vi "SaveTestTreeAs.vi"(7 "Action":T2, 8 "error in (no error)":errorcluster, 10 ".tst File Path":path, 11 "ListboxRef":refnum<vi>) -> (0 "error out":errorcluster, 1 "Cancelled?":bool, 2 "path.tstFile":path, 3 "All Test Tree Tags":string[](array[string]), 4 "Test Configuration":T1)   [LabVIEW 2018]
uses:
  TestConfigurationActions.ctl
  TestConfiguration.ctl
  <vilib>/Utility/config.llb/NI_LVConfig.lvlib
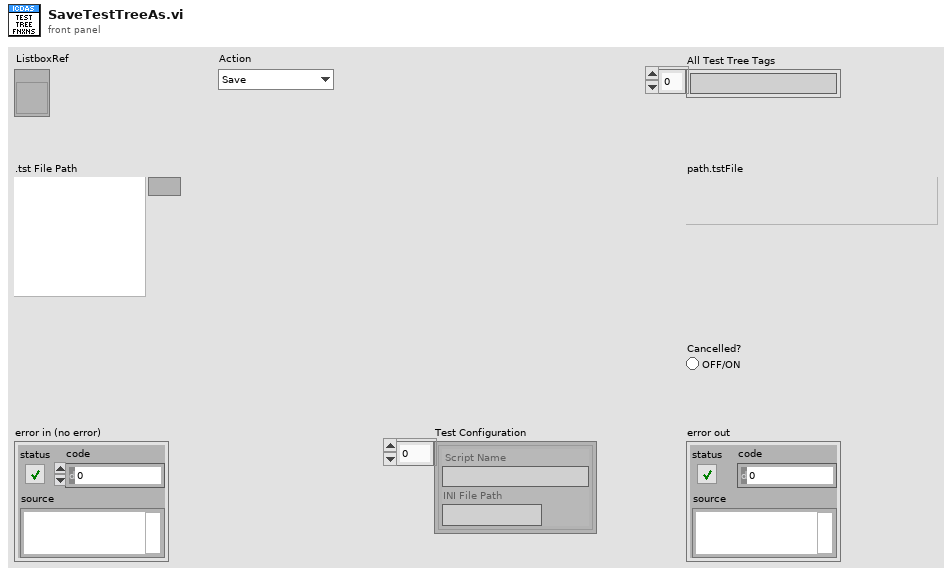
[diagram p1: front panel]
types:
  T1 = typedef "TestConfiguration.ctl" = cluster{"Script Name":string, "INI File Path":string}[]
  T2 = typedef "TestConfigurationActions.ctl" = enum16{"Save", "Save As", "Read", "Read&Load"}
  T3 = typedef "NI_LVConfig.lvlib/Config Data RefNum.ctl" = refnum<k1>
  T4 = typedef "cntlRefs.ctl" = cluster{"rngFGen":refnum<vi>, "rngDigitizer":refnum<vi>, "btnHide":refnum<vi>, "rngInst":refnum<vi>, "Instrument Modules":refnum<vi>, "RelativePathToINIFiles ":refnum<vi>, "PluginTree":refnum<vi>, "TestListboxRef":refnum<vi>, "path.tstFile":refnum<vi>, "cmbxRunningModules":refnum<vi>, "TestDataSubPanel":refnum<vi>, "TestDataCaption":refnum<vi>, "btnPopInOut":refnum<vi>, "PluginMgrQ":refnum<queue>, "TestMgrQ":refnum<queue>, "TestMgrSubPanel":refnum<vi>, "PluginMgrSubPanel":refnum<vi>, "PwrReqHandle":u32, "btnStopOneTest":refnum<vi>, "pathUserfiles":refnum<vi>}
  T5 = cluster{"Script Name":string, "INI File Path":string}
  T6 = typedef "Plugin Tree Tag.ctl" = cluster{"ItemType":T7, "Name":string, "Path":path, "Script":string[]}
  T7 = typedef "Plugins Tree Item Type.ctl" = enum16{"Plugin", "Instrument", "INI File", "INI Script"}
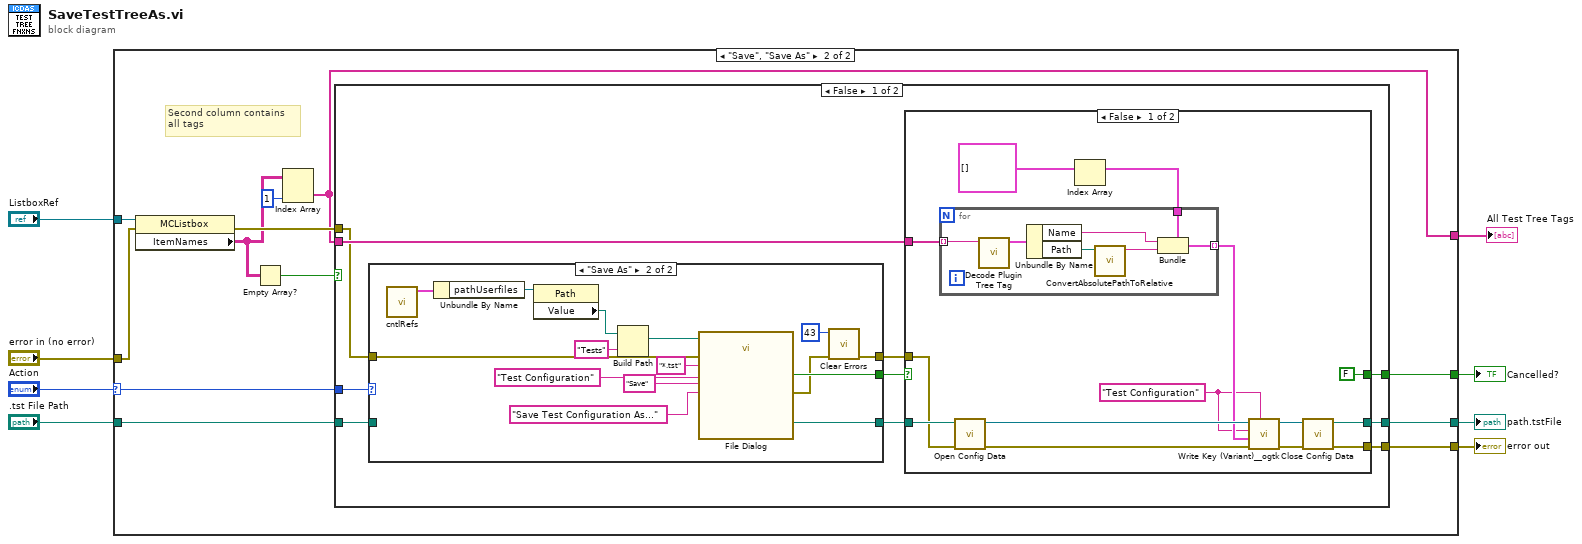
[diagram p0: block diagram]
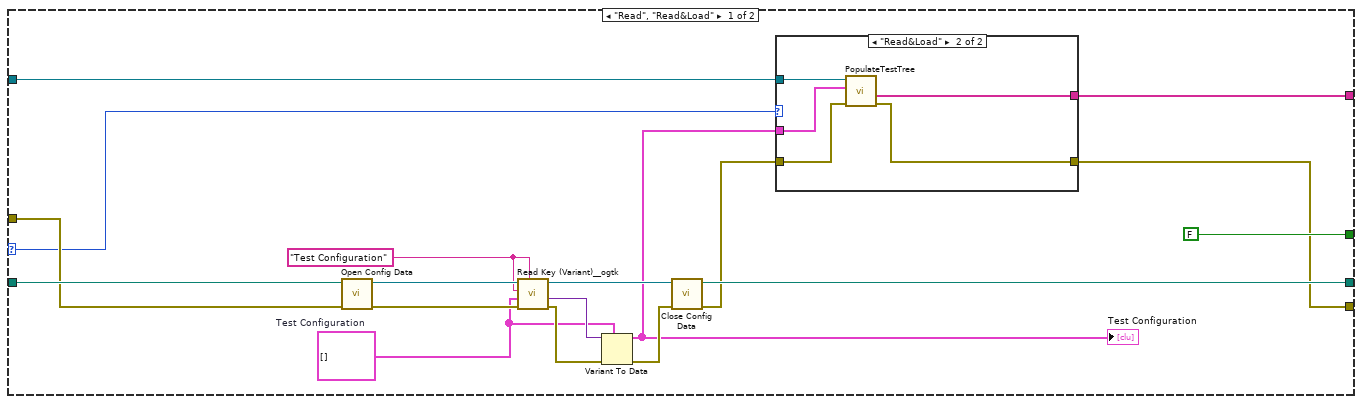
[diagram p2: hidden frame]
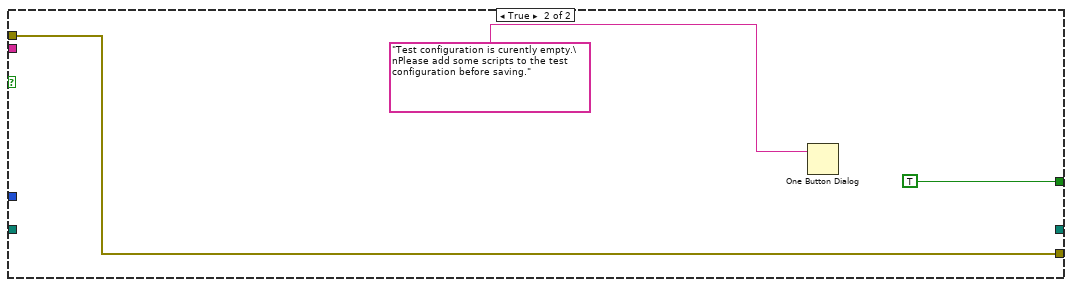
[diagram p6: hidden frame]
diagram:
  n1 = case shown="\"Save\", \"Save As\"" "Action" {
    selector: "Action" -> [w14 w40]
    tunnel: "ListboxRef" -> [w13 w43]
    tunnel: "error in (no error)" -> [w25 w42]
    tunnel: [w11 w39] -> w2
    tunnel: [FALSE w38] -> w5
    tunnel: [w18 w37] -> w4
    tunnel: ".tst File Path" -> [w26 w36]
    tunnel: [w9 w33] -> w1
    frame "Read", "Read&Load" {
      w15 = "Test Configuration" ("section")
      w21 = T1 []  # Test Configuration
      n2 = call <vilib>:"Open Config Data.vi"("error in (no error)"=w25, "configuration file path"=w26) -> ("error out"=w24:errorcluster, "refnum"=w16:T3)  [unwired: 7 in, 1 out]
      n3 = call <userlib>:"Read Key (Variant)__ogtk.vi"("section"=w15, "error in (no error)"=w24, "type"=w21, "key (optional)"=w15, "refnum"=w16) -> ("error out"=w22:errorcluster, "key-value"=w23:variant, "refnum out"=w19:T3)  [unwired: 3 in, 1 out]
      n4 = Variant To Data(error in=w22, type=w21, Variant=w23) -> (data=w10:T1, error out=w20:errorcluster)
      "Test Configuration" <- w10
      n5 = call <vilib>:"Close Config Data.vi"("error in (no error)"=w20, "refnum"=w19) -> ("error out"=w12:errorcluster, "file path"=w18:path)  [unwired: 8 in]
      n6 = case shown="\"Read&Load\"" w14 {
        tunnel: w13 -> [_ w32]
        tunnel: w10 -> [_ w31]
        tunnel: w12 -> [w27 w29]
        tunnel: [w27 w30] -> w11
        tunnel: [_ w28] -> w9
        frame Default {
        }
        frame "Read&Load" {
          n7 = call "PopulateTestTree.vi"("error in (no error)"=w29, "Test Configuration"=w31, "ListboxRef"=w32) -> ("error out"=w30:errorcluster, "All Test Tree Tags"=w28:string[])  [unwired: 7 in]
        }
      }
    }
    frame "Save", "Save As" {
      # "Second column contains\nall tags"
      n8 = property class="MCListbox"(reference=w43, error in=w42) -> (error out=w41:errorcluster, "ItemNames"=w34:string[][])  [unwired: 1 out]
      n9 = Empty Array?(array=w34) -> (empty?=w44:bool)
      n10 = Index Array(array=w34, index (col)=1 ("disabled index (col)")) -> (element=w33:string[])  [unwired: 1 in]
      n11 = case shown="False" w44 {
        tunnel: w33 -> [w54 _]
        tunnel: w41 -> [w53 w97]
        tunnel: w40 -> [w49 _]
        tunnel: [w48 w97] -> w39
        tunnel: [w47 _] -> w37
        tunnel: [w46 TRUE] -> w38
        tunnel: w36 -> [w45 _]
        frame False {
          n12 = case shown="\"Save As\"" w49 {
            tunnel: w53 -> [w56 w71]
            tunnel: [_ w70] -> w52
            tunnel: [w55 w69] -> w51
            tunnel: [w56 w58] -> w50
            tunnel: w45 -> [w55 _]
            frame "Save", Default {
            }
            frame "Save As" {
              n13 = call "cntlRefs.vi"() -> ("cntlRefs"=w61:T4)  [unwired: 10 in, 1 out]
              n14 = Unbundle By Name(w61) -> ("pathUserfiles"=w60:refnum<vi>)
              n15 = property class="Path"(reference=w60) -> ("Value"=w59:path)  [unwired: 1 in, 2 out]
              n16 = Build Path(base path=w59, name or relative path="Tests") -> (appended path=w65:path)
              n17 = call "File Dialog"("start path"=w65, "prompt"="Save Test Configuration As...", "button label"="Save", "error in"=w71, "pattern (all files)"="*.tst", "pattern label"="Test Configuration") -> ("selected path"=w69:path, "cancelled"=w70:bool, "error out"=w68:errorcluster)  [unwired: 6 in, 1 out]
              n18 = call <vilib>:"Clear Errors.vi"("error in (no error)"=w68, "specific error code to clear (0: all)"=43) -> ("error out"=w58:errorcluster)  [unwired: 4 in, 1 out]
            }
          }
          n19 = case shown="False" w52 {
            selector: w52 -> [_ w93]
            tunnel: w54 -> [w85 _]
            tunnel: w51 -> [w83 w94]
            tunnel: w50 -> [w82 w95]
            tunnel: [w75 w95] -> w48
            tunnel: [w74 w94] -> w47
            tunnel: [FALSE w93] -> w46
            frame False {
              w78 = "Test Configuration" ("section")
              n20 = call <vilib>:"Open Config Data.vi"("error in (no error)"=w82, "configuration file path"=w83) -> ("error out"=w80:errorcluster, "refnum"=w81:T3)  [unwired: 7 in, 1 out]
              n21 = Index Array(array=T1 [] ("Test Configuration")) -> (element=w72:T5)  [unwired: 1 in]
              n22 = for {
                tunnel: w85 -> [w92] mode=indexing
                tunnel: w72 -> [w89]
                tunnel: [w86] -> w79 mode=indexing
                n23 = call "Decode Plugin Tree Tag.vi"("Tag"=w92) -> ("Plugin Tree Tag"=w91:T6)  [unwired: 9 in, 1 out]
                n24 = Unbundle By Name(w91) -> ("Name"=w87:string, "Path"=w90:path)
                n25 = call "ConvertAbsolutePathToRelative.vi"("Absolute Path"=w90) -> ("RelativePath"=w88:string)  [unwired: 10 in]
                n26 = Bundle(cluster=w89, "Script Name"=w87, "INI File Path"=w88) -> (w86:T5)
              }
              n27 = call <userlib>:"Write Key (Variant)__ogtk.vi"("section"=w78, "error in (no error)"=w80, "key-value"=w79, "key (optional)"=w78, "refnum"=w81) -> ("error out"=w77:errorcluster, "refnum out"=w76:T3)  [unwired: 5 in]
              n28 = call <vilib>:"Close Config Data.vi"("error in (no error)"=w77, "refnum"=w76) -> ("error out"=w75:errorcluster, "file path"=w74:path)  [unwired: 8 in]
            }
            frame True {
            }
          }
        }
        frame True {
          n29 = One Button Dialog(message="Test configuration is curently empty.\nPlease add some scripts to the test configuration before saving.") -> ()  [unwired: 1 in, 1 out]
        }
      }
    }
  }
  "error out" <- w2
  "Cancelled?" <- w5
  "path.tstFile" <- w4
  "All Test Tree Tags" <- w1
